vi "onAssertionSlippage.vi"(7 "AssertEqualValue in":refnum<class "AssertEqualValue.lvclass">, 10 "Properties":refnum<class "Properties.Assert.lvclass">) -> (0 "error out":errorcluster, 2 "Properties out":refnum<class "Properties.Assert.lvclass">)   [LabVIEW 2021, in "Bananas.lvlib" / "AssertEqualValue.lvclass"]
uses:
  AssertEqualValue.lvclass
  <vilib>/addons/_JKI Toolkits/Caraya/classes/Properties.Assert/Properties.Assert.lvclass
  C:/Program Files (x86)/National Instruments/LabVIEW 2021/vi.lib/addons/_JKI Toolkits/Caraya/classes/Properties/Properties.lvclass
  <vilib>/addons/_JKI Toolkits/Caraya/classes/Properties.Assert/Properties.Assert.lvclass/Properties.Assert.ctl
  AssertEqualValue.lvclass/AssertEqualValue.ctl
  Read Y.vi
  Read X.vi
  <vilib>/addons/_JKI Toolkits/Caraya/classes/Properties/Properties.lvclass
  Bananas.lvlib
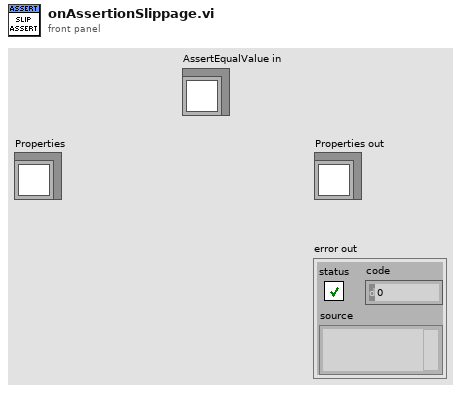
[diagram p1: front panel]
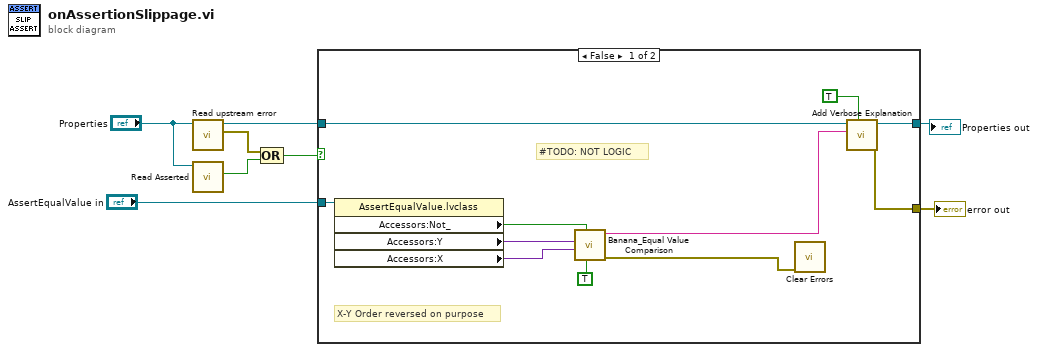
[diagram p0: block diagram]
diagram:
  n1 = call <vilib>:"Read upstream error.vi"("Properties.Assert in"="Properties") -> ("upstream-error"=w7:errorcluster, "Properties.Assert out"=w8:refnum<class "Properties.Assert.lvclass">)  [unwired: 9 in]
  n2 = call <vilib>:"Read Asserted.vi"("Properties.Assert in"="Properties") -> ("Asserted"=w6:bool)  [unwired: 9 in, 1 out]
  n3 = Compound Arithmetic op=OR(w7, w6) -> (w5:bool)
  n4 = case shown="False" w5 {
    tunnel: [w18 w20] -> w3
    tunnel: [w17 _] -> w2
    tunnel: w8 -> [w19 w20]
    tunnel: "AssertEqualValue in" -> [w15 _]
    frame False {
      # "X-Y Order reversed on purpose"
      # "#TODO: NOT LOGIC"
      n5 = property class="AssertEqualValue.lvclass"(reference=w15) -> ("Accessors:Not_"=w9:bool, "Accessors:Y"=w14:variant, "Accessors:X"=w13:variant)  [unwired: 1 in, 2 out]
      n6 = call "Banana_Equal Value Comparison.vi"("verbose? (F)"=TRUE, "Not? (F)"=w9, "Y"=w13, "X"=w14) -> ("error out"=w10:errorcluster, "Verbose output"=w12:string)  [unwired: 5 in, 1 out]
      n7 = call <vilib>:"Clear Errors.vi"("error in (no error)"=w10) -> ()  [unwired: 5 in, 2 out]
      n8 = call <vilib>:"Add Verbose Explanation.vi"("overwrite?"=TRUE, "Verbose Explanation"=w12, "Properties"=w19) -> ("error out"=w17:errorcluster, "Properties"=w18:refnum<class "Properties.Assert.lvclass">)  [unwired: 7 in]
    }
    frame True {
      # "There was an upstream error or the assertion = TRUE"
    }
  }
  "error out" <- w2
  "Properties out" <- w3
